vi "hit himself.vi"(8 "error in (no error)":errorcluster, 11 "Board_Game in":refnum<class "Board_Game.lvclass">) -> (0 "error out":errorcluster, 2 "HIT":bool, 3 "Board_Game out":refnum<class "Board_Game.lvclass">)   [LabVIEW 2021, in "Board_Game.lvclass"]
uses:
  Board_Game.lvclass
  Board_Game.lvclass/Board_Game.ctl
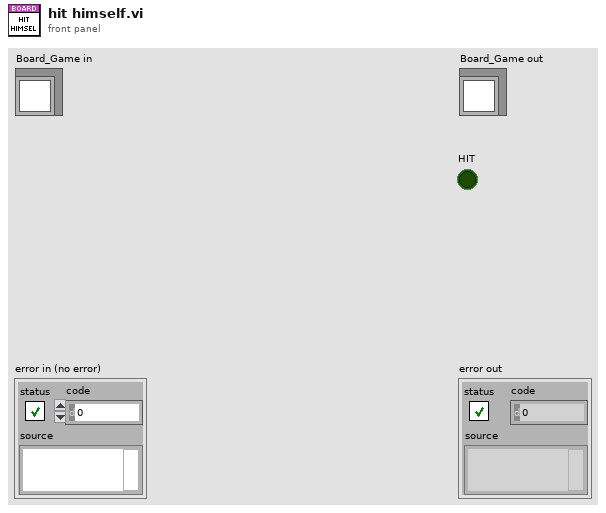
[diagram p1: front panel]
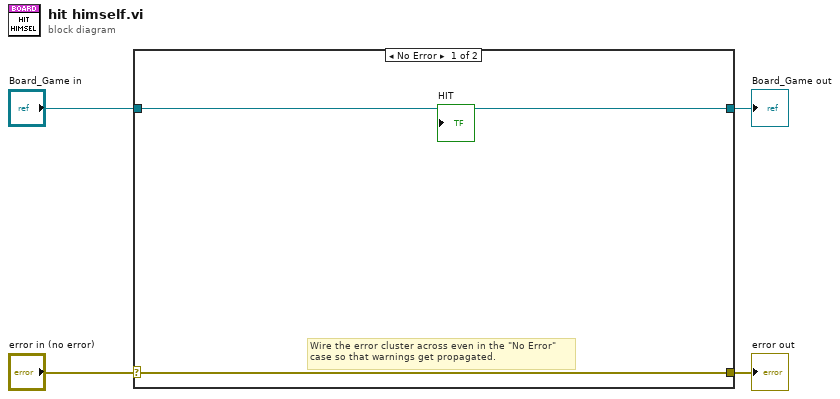
[diagram p0: block diagram]
diagram:
  n1 = case shown="No Error" "error in (no error)" {
    selector: "error in (no error)" -> [w5 w8]
    tunnel: [w5 w8] -> w3
    tunnel: [w6 w7] -> w1
    tunnel: "Board_Game in" -> [w6 w7]
    frame No Error {
      # "Wire the error cluster across even in the \"No Error\"\ncase so that warnings get propagated."
    }
    frame Error {
    }
  }
  "error out" <- w3
  "Board_Game out" <- w1
